vi "Open Key.vi"(7 "Crypto Provider":T1, 8 "error in (no error)":errorcluster, 11 "Key Name":string) -> (0 "error out":errorcluster, 3 "CngKey out":refnum<k24>)   [LabVIEW 2021, in "dotNET Crypto Key Management.lvlib"]
uses:
  dotNET Crypto Key Management.lvlib
  CNG Provider Type.ctl
  System.Core
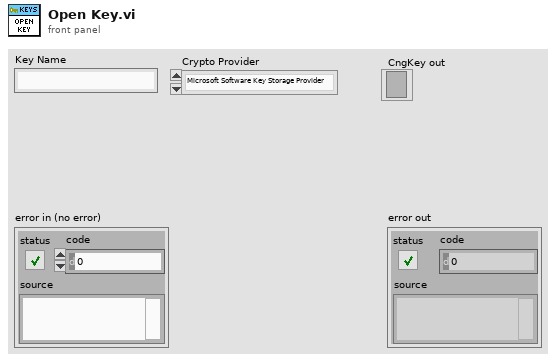
[diagram p1: front panel]
types:
  T1 = typedef "dotNET Crypto Key Management.lvlib/CNG Provider Type.ctl" = enum16{"Microsoft Software Key Storage Provider", "Microsoft Platform Crypto Provider"}
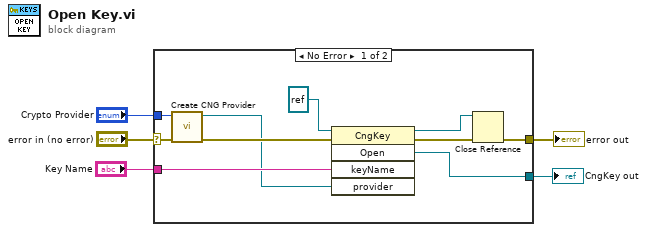
[diagram p0: block diagram]
diagram:
  n1 = case shown="No Error" "error in (no error)" {
    selector: "error in (no error)" -> [w13 w16]
    tunnel: "Crypto Provider" -> [w11 _]
    tunnel: "Key Name" -> [w10 _]
    tunnel: [w8 w16] -> w2
    tunnel: [w6 _] -> w1
    frame No Error {
      n2 = call "Create CNG Provider.vi"("error in (no error)"=w13, "Crypto Provider"=w11) -> ("error out"=w12:errorcluster, "CngProvider"=w9:refnum<k24>)  [unwired: 8 in]
      n3 = invoke class="CngKey" method="Open"(reference=refnum<k24> refnum, error in=w12, "keyName"=w10, "provider"=w9) -> (reference out=w7:refnum<k24>, error out=w14:errorcluster, "Open"=w6:refnum<k24>)  [unwired: 1 in, 2 out]
      n4 = Close Reference(reference=w7, error in (no error)=w14) -> (error out=w8:errorcluster)
    }
    frame Error {
    }
  }
  "error out" <- w2
  "CngKey out" <- w1
